vi "File2.List All Files in a Directory Tree.vi"(8 "error in (no error)":errorcluster, 11 "Folder":path) -> (0 "error out":errorcluster, 3 "Files":path[](array[path]))   [LabVIEW 2024]
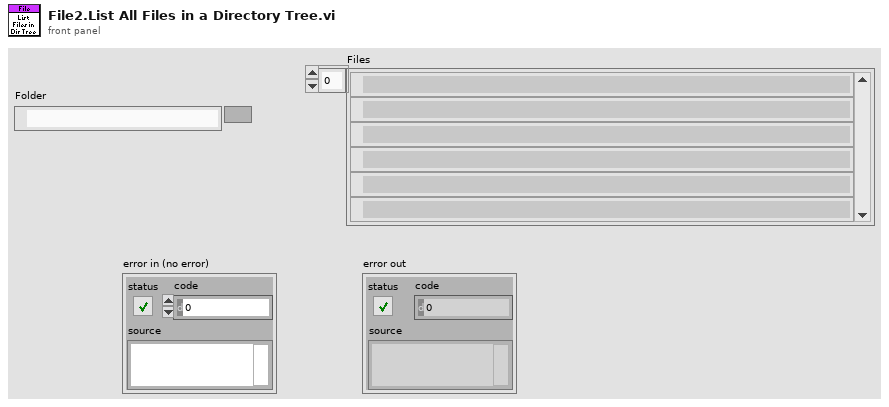
[diagram p1: front panel]
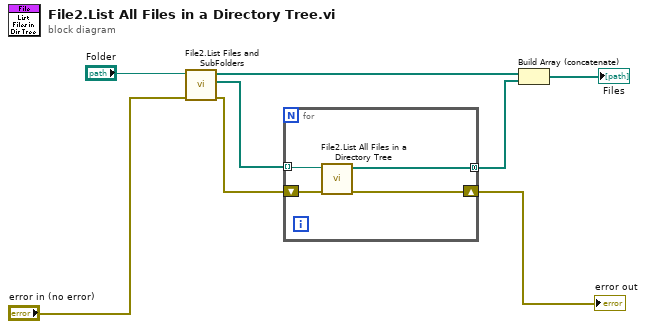
[diagram p0: block diagram]
diagram:
  n1 = call "File2.List Files and SubFolders.vi"("error in (no error)"="error in (no error)", "Folder"="Folder") -> ("error out"=w2:errorcluster, "Folders"=w7:path[], "Files"=w6:path[])  [unwired: 7 in]
  n2 = for {
    tunnel: w7 -> [w12] mode=indexing
    tunnel: [w11] -> w5 mode=concatenating
    shift-right: [w9] -> w1
    shift-left: w2 -> [w10]
    n3 = call "File2.List All Files in a Directory Tree.vi"("error in (no error)"=w10, "Folder"=w12) -> ("error out"=w9:errorcluster, "Files"=w11:path[])  [unwired: 8 in]
  }
  "error out" <- w1
  n4 = Build Array (concatenate)(w6, w5) -> (→"Files":path[])
